vi "Q8381 Axis Unit Display.vi"(2 "LOSS Measure?":bool, 3 "Y Input":dbl format="%.2f") -> (0 "Y unit":string, 1 "Data Error":bool)   [LabVIEW 2017]
doc: "Displays Reference Level unit. They are dBm, mW, uW or nW. If Loss is measured, the unit will be dB."
panel:
  out "Y Magnitude":string
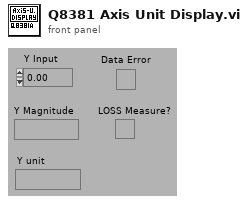
[diagram p1: front panel]
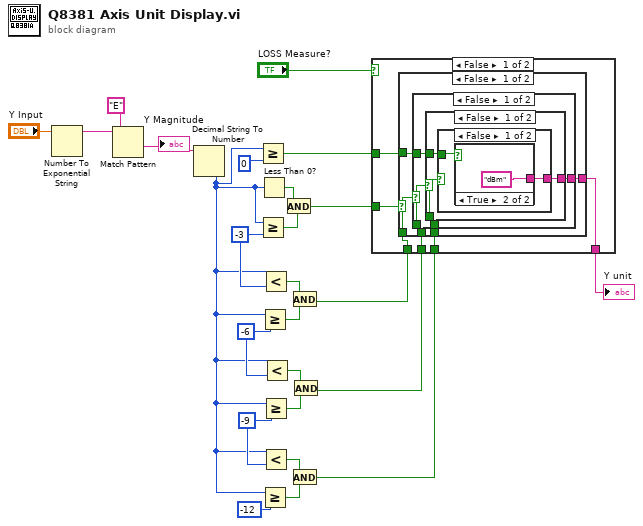
[diagram p0: block diagram]
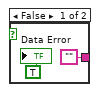
[diagram p2: hidden frame]
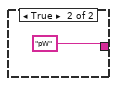
[diagram p3: hidden frame]
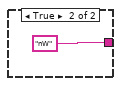
[diagram p4: hidden frame]
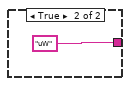
[diagram p5: hidden frame]
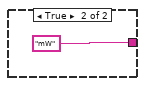
[diagram p6: hidden frame]
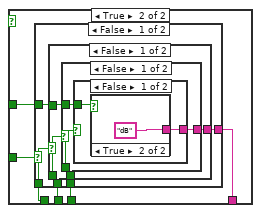
[diagram p7: hidden frame]
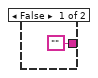
[diagram p8: hidden frame]
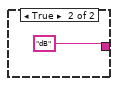
[diagram p9: hidden frame]
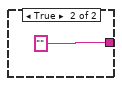
[diagram p10: hidden frame]
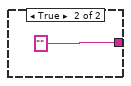
[diagram p11: hidden frame]
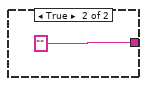
[diagram p12: hidden frame]
diagram:
  w13 = -9
  w20 = -6
  w21 = -3
  n1 = Number To Exponential String(number="Y Input") -> (E-format string=w24:string)  [unwired: 3 in]
  n2 = Match Pattern(string=w24, regular expression="E") -> (after substring=w22:string)  [unwired: 1 in, 3 out]
  "Y Magnitude" <- w22
  n3 = Decimal String To Number(string=w22) -> (number=w2:i32)  [unwired: 2 in, 1 out]
  n4 = Greater Or Equal?(x=w2, y=0) -> (x >= y?=w8:bool)
  n5 = Greater Or Equal?(x=w2, y=w21) -> (x >= y?=w15:bool)
  n6 = Less Than 0?(x=w2) -> (x < 0?=w16:bool)
  n7 = Greater Or Equal?(x=w2, y=w20) -> (x >= y?=w18:bool)
  n8 = Greater Or Equal?(x=w2, y=-12) -> (x >= y?=w5:bool)
  n9 = Less?(x=w2, y=w21) -> (x < y?=w19:bool)
  n10 = Greater Or Equal?(x=w2, y=w13) -> (x >= y?=w11:bool)
  n11 = Less?(x=w2, y=w13) -> (x < y?=w6:bool)
  n12 = Less?(x=w2, y=w20) -> (x < y?=w12:bool)
  n13 = And(x=w16, y=w15) -> (x .and. y?=w17:bool)
  n14 = And(x=w19, y=w18) -> (x .and. y?=w14:bool)
  n15 = And(x=w6, y=w5) -> (x .and. y?=w4:bool)
  n16 = And(x=w12, y=w11) -> (x .and. y?=w10:bool)
  n17 = case shown="False" "LOSS Measure?" {
    tunnel: w4 -> [w31 w54]
    tunnel: w8 -> [w30 w58]
    tunnel: w10 -> [w29 w55]
    tunnel: w14 -> [w28 w56]
    tunnel: w17 -> [w27 w57]
    tunnel: [w26 w53] -> w1
    frame False {
      n18 = case shown="False" w27 {
        tunnel: [w35 "mW"] -> w26
        tunnel: w28 -> [w36 _]
        tunnel: w29 -> [w34 _]
        tunnel: w30 -> [w33 _]
        tunnel: w31 -> [w32 _]
        frame False {
          n19 = case shown="False" w36 {
            tunnel: [w39 "uW"] -> w35
            tunnel: w34 -> [w40 _]
            tunnel: w33 -> [w38 _]
            tunnel: w32 -> [w37 _]
            frame False {
              n20 = case shown="False" w40 {
                tunnel: [w43 "nW"] -> w39
                tunnel: w38 -> [w41 _]
                tunnel: w37 -> [w42 _]
                frame False {
                  n21 = case shown="False" w42 {
                    tunnel: [w45 "pW"] -> w43
                    tunnel: w41 -> [w44 _]
                    frame False {
                      n22 = case shown="True" w44 {
                        tunnel: ["" "dBm"] -> w45
                        frame False {
                          "Data Error" <- TRUE
                        }
                        frame True {
                        }
                      }
                    }
                    frame True {
                    }
                  }
                }
                frame True {
                }
              }
            }
            frame True {
            }
          }
        }
        frame True {
        }
      }
    }
    frame True {
      n23 = case shown="False" w57 {
        tunnel: [w62 ""] -> w53
        tunnel: w56 -> [w63 _]
        tunnel: w55 -> [w61 _]
        tunnel: w58 -> [w60 _]
        tunnel: w54 -> [w59 _]
        frame False {
          n24 = case shown="False" w63 {
            tunnel: [w66 ""] -> w62
            tunnel: w61 -> [w67 _]
            tunnel: w60 -> [w65 _]
            tunnel: w59 -> [w64 _]
            frame False {
              n25 = case shown="False" w67 {
                tunnel: [w70 ""] -> w66
                tunnel: w65 -> [w68 _]
                tunnel: w64 -> [w69 _]
                frame False {
                  n26 = case shown="False" w69 {
                    tunnel: [w72 "dB"] -> w70
                    tunnel: w68 -> [w71 _]
                    frame False {
                      n27 = case shown="True" w71 {
                        tunnel: ["" "dB"] -> w72
                        frame False {
                        }
                        frame True {
                        }
                      }
                    }
                    frame True {
                    }
                  }
                }
                frame True {
                }
              }
            }
            frame True {
            }
          }
        }
        frame True {
        }
      }
    }
  }
  "Y unit" <- w1
